vi "set Voxel Dimensions In Real Units.vi"(7 "pVoxelDepthInRealUnits":dbl, 8 "error in (no error)":errorcluster, 9 "pVoxelHeightInRealUnits":dbl, 10 "pVoxelWidthInRealUnits":dbl, 11 "pSinkId":i32) -> (0 "error out":errorcluster, 3 "function return":i32)   [LabVIEW 2012, in "clearvolume.lvlib"]
doc: "__declspec(dllexport) long __cdecl setVoxelDimensionsInRealUnits( long pSinkId,\n double pVoxelWidthInRealUnits,\n double pVoxelHeightInRealUnits,\n double pVoxelDepthInRealUnits);"
uses:
  clearvolume.lvlib
  clearvolume.dll
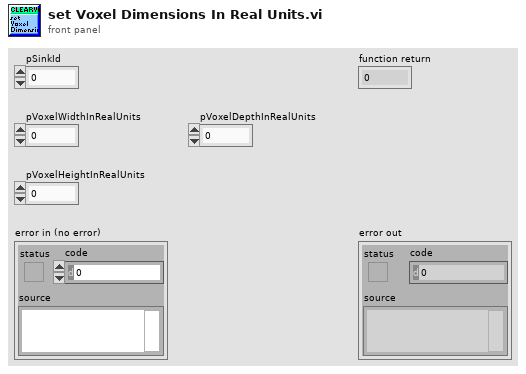
[diagram p1: front panel]
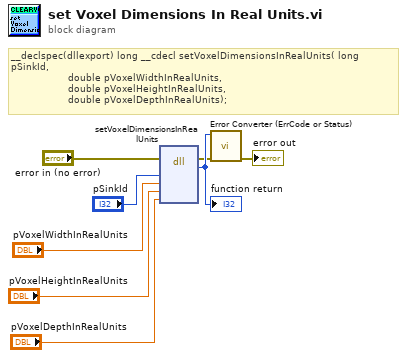
[diagram p0: block diagram]
diagram:
  # "__declspec(dllexport) long __cdecl setVoxelDimensionsInRealUnits( long pSinkId,\n\t\t\t\t\t\t\t\t\t\t\t\t\t\t\t\t\t\t\tdouble pVoxelWidthInRealUnits,\n\t\t\t\t\t\t\t\t\t\t\t\t\t\t\t\t\t\t\tdouble pVoxelHeightInRealUnits,\n\t\t\t\t\t\t\t\t\t\t\t\t\t\t\t\t\t\t\tdouble pVoxelDepthInRealUnits);"
  n1 = dll-call lib="C:/Users/myerslab/workspace/Libraries/CV/clearvolume/src/labview/clearvolume/clearvolume.*" fn="setVoxelDimensionsInRealUnits"(error in="error in (no error)", "pSinkId"="pSinkId", "pVoxelWidthInRealUnits"="pVoxelWidthInRealUnits", "pVoxelHeightInRealUnits"="pVoxelHeightInRealUnits", "pVoxelDepthInRealUnits"="pVoxelDepthInRealUnits") -> (error out=w2:errorcluster, w8:i32)  [unwired: 6 in, 1 out]
  "function return" <- w8
  n2 = call "Error Converter (ErrCode or Status).vi"("error in (no error)"=w2, "error code"=w8) -> ("error out"=→"error out":errorcluster)  [unwired: 9 in]
